vi "CAN_DEBUG_Send.vi"() -> ()   [LabVIEW 2011]
uses:
  _USB_CAN_GLOBAL_.vi
  <vilib>/Utility/file.llb/Read From Spreadsheet File (string).vi
panel:
  in  "channel":u16(ring) items=["通道0", "通道1"]
  in  "TFun":u32
  in  "remote":bool
  in  "ExtFrame":bool
  in  "event":refnum<user-event>
  in  "sendfile":bool
  in  "ID":u32
  in  "Enable":bool
  in  "stop":bool
  in  "Data Inc":bool
  in  "ID Inc":bool
  in  "Cycle":i32=10
  in  "FrameCnt":i32
  in  "data":u8[](array[numeric]) format="%02x"
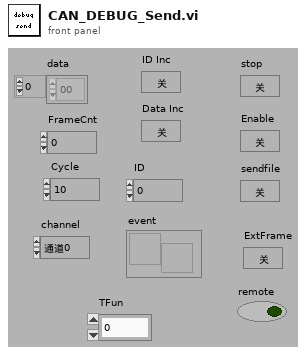
[diagram p1: front panel]
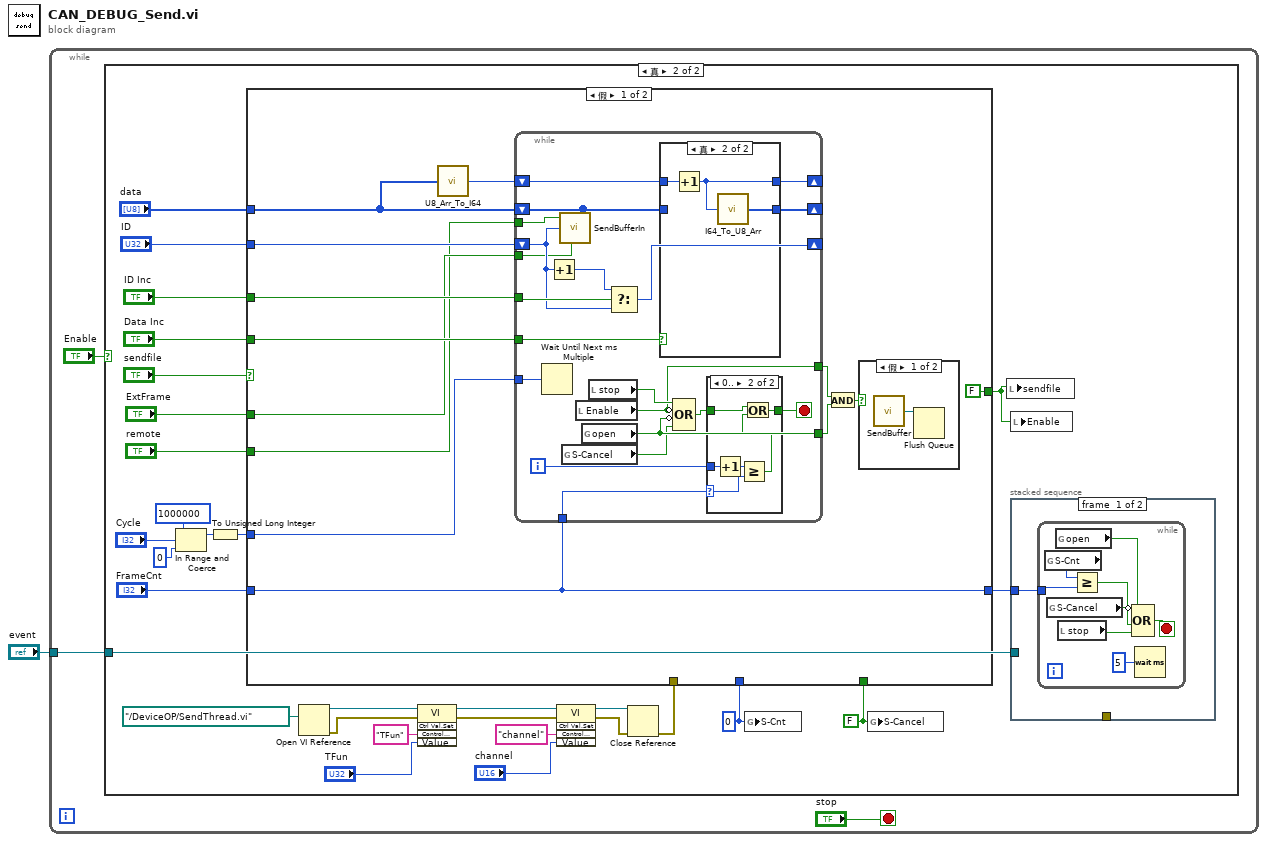
[diagram p0: block diagram]
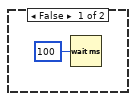
[diagram p2: hidden frame]
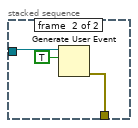
[diagram p3: hidden frame]
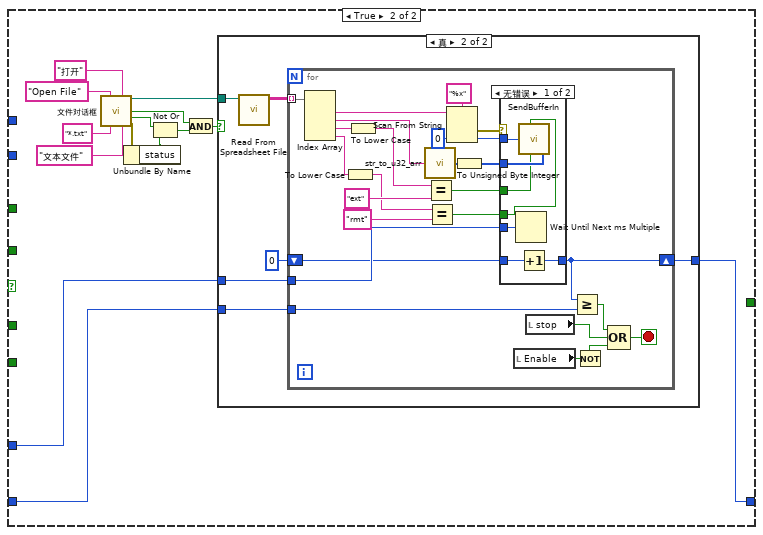
[diagram p7: hidden frame]
diagram:
  n1 = while {
    tunnel: "event" -> [w2]
    stop <- "stop" stop-if-true
    n2 = case shown="真" "Enable" {
      tunnel: w2 -> [_ w14]
      frame False {
        n3 = Wait (ms)(milliseconds to wait=u32 100 ("等待时间（毫秒）")) -> ()  [unwired: 1 out]
      }
      frame True {
        w13 = FALSE ("S-Cancel")
        w17 = u32 0 ("S-Cnt")
        n4 = In Range and Coerce(upper limit=1000000 ("上限"), x="Cycle", lower limit=0 ("下限")) -> (coerced(x)=w30:i32)  [unwired: 1 out]
        n5 = To Unsigned Long Integer(number=w30) -> (unsigned 32bit integer=w29:u32)
        n6 = Open VI Reference(vi path=path "../DeviceOP/SendThread.vi" ("VI路径")) -> (vi reference=w22:refnum<vi>, error out=w21:errorcluster)  [unwired: 5 in]
        n7 = invoke class="VI" method="Ctrl Val.Set"(reference=w22, error in=w21, "Control Name"="TFun" ("控件名"), "Value"="TFun") -> (reference out=w12:refnum<vi>, error out=w11:errorcluster)  [unwired: 1 in, 3 out]
        n8 = invoke class="VI" method="Ctrl Val.Set"(reference=w12, error in=w11, "Control Name"="channel" ("控件名"), "Value"="channel") -> (reference out=w10:refnum<vi>, error out=w9:errorcluster)  [unwired: 1 in, 3 out]
        n9 = Close Reference(reference=w10, error in (no error)=w9) -> (error out=w18:errorcluster)
        n10 = case shown="假" "sendfile" {
          tunnel: "FrameCnt" -> [w53 w96]
          tunnel: w29 -> [w54 w95]
          tunnel: "data" -> [w49 _]
          tunnel: "ID" -> [w60 _]
          tunnel: "ID Inc" -> [w59 _]
          tunnel: "Data Inc" -> [w58 _]
          tunnel: [FALSE ("Enable") _] -> w16
          tunnel: "ExtFrame" -> [w56 _]
          tunnel: "remote" -> [w55 _]
          tunnel: w18 -> [_ _]
          tunnel: w17 -> [_ _]
          tunnel: [w53 w94] -> w15
          tunnel: w13 -> [_ _]
          frame False {
            n11 = call "U8_Arr_To_I64.vi"("data"=w49) -> ("I64"=w48:i64)
            n12 = while {
              shift-right: [w73] -> _
              shift-left: w49 -> [w74]
              shift-right: [w76] -> _
              shift-left: w60 -> [w77]
              tunnel: w59 -> [w79]
              tunnel: w58 -> [w75]
              tunnel: w54 -> [w80]
              shift-right: [w71] -> _
              shift-left: w48 -> [w72]
              tunnel: w56 -> [w69]
              tunnel: w55 -> [w68]
              tunnel: [w67] -> w51
              tunnel: w53 -> [w66]
              tunnel: [w62] -> w52
              i -> [w63]
              stop <- w64 stop-if-true
              n13 = Wait Until Next ms Multiple(millisecond multiple=w80) -> ()  [unwired: 1 out]
              n14 = Increment(x=w77) -> (x+1=w78:u32)
              n15 = call "SendBufferIn.vi"("remote"=w68, "ID"=w77, "ExtFrame"=w69, "数据"=w74) -> ()  [unwired: 2 in]
              n16 = global read "_USB_CAN_GLOBAL_.vi" "S-Cancel"() -> (w61:bool)
              n17 = local read "Enable"() -> (w62:bool)
              n18 = global read "_USB_CAN_GLOBAL_.vi" "open"() -> (w67:bool)
              n19 = local read "stop"() -> (w70:bool)
              n20 = Select(t=w78, s=w79, f=w77) -> (s? t:f=w76:u32)
              n21 = case shown="真" w75 {
                tunnel: w74 -> [w89 _]
                tunnel: [w89 w91] -> w73
                tunnel: w72 -> [w88 w92]
                tunnel: [w88 w90] -> w71
                frame False {
                }
                frame True {
                  n22 = Increment(x=w92) -> (x+1=w90:i64)
                  n23 = call "I64_To_U8_Arr.vi"("U64"=w90) -> ("data"=w91:u8[])
                }
              }
              n24 = Compound Arithmetic op=OR(w70, invert w62, invert w67, w61) -> (w65:bool)
              n25 = case shown="0.." w66 {
                selector: w66 -> [_ w85]
                tunnel: w65 -> [w81 w83]
                tunnel: [w81 w84] -> w64
                tunnel: w63 -> [_ w87]
                frame -1, Default {
                }
                frame 0.. {
                  n26 = Increment(x=w87) -> (x+1=w86:i32)
                  n27 = Greater Or Equal?(x=w86, y=w85) -> (x >= y?=w82:bool)
                  n28 = Or(x=w83, y=w82) -> (x .or. y?=w84:bool)
                }
              }
            }
            n29 = And(x=w52, y=w51) -> (x .and. y?=w50:bool)
            n30 = case shown="假" w50 {
              frame False {
                n31 = call "SendBuffer.vi"() -> ("VCI_CAN_BUF_T"=w93:refnum<queue>)  [unwired: 1 in]
                n32 = Flush Queue(queue=w93) -> ()  [unwired: 1 in, 3 out]
              }
              frame True {
              }
            }
          }
          frame True {
            n33 = call "文件对话框"("prompt"="Open File", "button label"="打开", "pattern (all files)"="*.txt", "pattern label"="文本文件") -> ("selected path"=w97:path, "exists"=w99:bool, "cancelled"=w101:bool, "error out"=w103:errorcluster)  [unwired: 8 in]
            n34 = Unbundle By Name(w103) -> ("status"=w102:bool)
            n35 = Not Or(1:w102, 2:w101) -> (0:w100:bool)
            n36 = And(x=w99, y=w100) -> (x .and. y?=w98:bool)
            n37 = case shown="真" w98 {
              tunnel: w97 -> [_ w113]
              tunnel: w96 -> [_ w110]
              tunnel: w95 -> [_ w112]
              tunnel: [_ w108] -> w94
              frame False {
              }
              frame True {
                n38 = call-poly <vilib>:"Read From Spreadsheet File.vi"("file path (dialog if empty)"=w113) -> ("all rows"=w111:string[][])  [unwired: 6 in, 4 out]
                n39 = for {
                  tunnel: w111 -> [w139] mode=indexing
                  tunnel: w112 -> [w130]
                  tunnel: w110 -> [w115]
                  shift-right: [w116] -> w108
                  shift-left: 0 -> [w117]
                  stop <- w127 stop-if-true
                  n40 = Index Array(array=w139) -> (element #1=w138:string, element #2=w135:string, element #3=w125:string, element #4=w122:string)  [unwired: 4 in]
                  n41 = To Lower Case(string=w122) -> (all lower case string=w119:string)
                  n42 = To Lower Case(string=w125) -> (all lower case string=w120:string)
                  n43 = call "str_to_u32_arr.vi"("string"=w135) -> ("array"=w134:u32[])
                  n44 = Equal?(x=w120, y="ext") -> (x = y?=w124:bool)
                  n45 = Equal?(x=w119, y="rmt") -> (x = y?=w118:bool)
                  n46 = Scan From String(format string="%x" ("格式字符串"), input string=w138, default 1=u32 0) -> (error out=w133:errorcluster, output 1=w132:u32)  [unwired: 2 in, 2 out]
                  n47 = To Unsigned Byte Integer(number=w134) -> (unsigned 8bit integer=w131:u8[])
                  n48 = case shown="无错误" w133 {
                    tunnel: w132 -> [w146 _]
                    tunnel: w131 -> [w145 _]
                    tunnel: w130 -> [w144 _]
                    tunnel: w124 -> [w143 _]
                    tunnel: w118 -> [w142 _]
                    tunnel: w117 -> [w141 w147]
                    tunnel: [w140 w147] -> w116
                    frame No Error {
                      n49 = Wait Until Next ms Multiple(millisecond multiple=w144) -> ()  [unwired: 1 out]
                      n50 = call "SendBufferIn.vi"("remote"=w142, "ID"=w146, "ExtFrame"=w143, "数据"=w145) -> ()  [unwired: 2 in]
                      n51 = Increment(x=w141) -> (x+1=w140:i32)
                    }
                    frame Error {
                    }
                  }
                  n52 = local read "Enable"() -> (w128:bool)
                  n53 = local read "stop"() -> (w129:bool)
                  n54 = Greater Or Equal?(x=w116, y=w115) -> (x >= y?=w114:bool)
                  n55 = Not(x=w128) -> (.not. x?=w126:bool)
                  n56 = Compound Arithmetic op=OR(w114, w129, w126) -> (w127:bool)
                }
              }
            }
          }
        }
        n57 = global write "_USB_CAN_GLOBAL_.vi" "S-Cnt"(w17) -> ()
        n58 = global write "_USB_CAN_GLOBAL_.vi" "S-Cancel"(w13) -> ()
        n59 = local write "sendfile"(w16) -> ()
        n60 = local write "Enable"(w16) -> ()
        n61 = stacked-sequence {
          tunnel: w15 -> [w36 _]
          tunnel: w14 -> [_ w47]
          tunnel: [_ w45] -> _
          frame #0 {
            n62 = while {
              tunnel: w36 -> [w43]
              stop <- w39 stop-if-true
              n63 = global read "_USB_CAN_GLOBAL_.vi" "S-Cnt"() -> (w42:i64)
              n64 = global read "_USB_CAN_GLOBAL_.vi" "S-Cancel"() -> (w38:bool)
              n65 = global read "_USB_CAN_GLOBAL_.vi" "open"() -> (w37:bool)
              n66 = local read "stop"() -> (w41:bool)
              n67 = Greater Or Equal?(x=w42, y=w43) -> (x >= y?=w40:bool)
              n68 = Compound Arithmetic op=OR(invert w37, w38, w40, w41) -> (w39:bool)
              n69 = Wait (ms)(milliseconds to wait=u32 5 ("等待时间（毫秒）")) -> ()  [unwired: 1 out]
            }
          }
          frame #1 {
            n70 = Generate User Event(user event=w47, event data cluster=TRUE ("事件数据")) -> (error out=w45:errorcluster)  [unwired: 1 in, 1 out]
          }
        }
      }
    }
  }
